vi "picoquant_read_buffer.vi"(8 "error in (no error)":errorcluster, 11 "picoquant_generic in":refnum<class "picoquant_generic.lvclass">) -> (0 "error out":errorcluster, 2 "new_data":u32[](array[numeric]), 3 "picoquant_generic out":refnum<class "picoquant_generic.lvclass">)   [LabVIEW 2015, in "picoquant_generic.lvclass"]
uses:
  picoquant_generic.lvclass
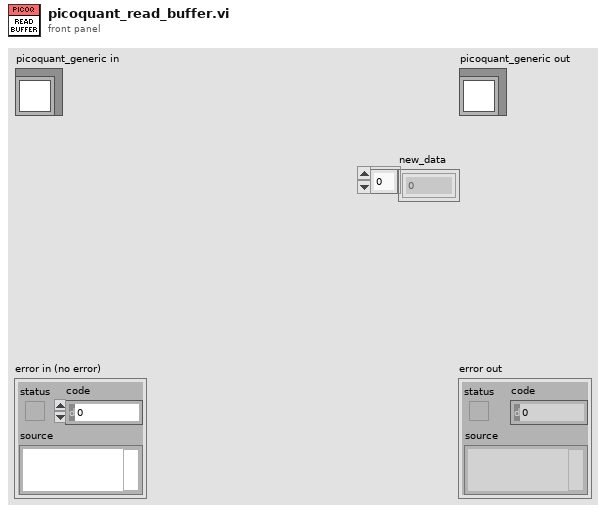
[diagram p1: front panel]
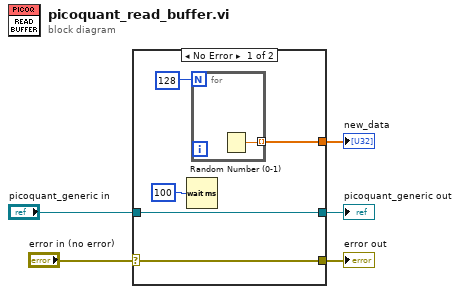
[diagram p0: block diagram]
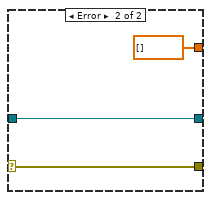
[diagram p2: hidden frame]
diagram:
  n1 = case shown="No Error" "error in (no error)" {
    selector: "error in (no error)" -> [w9 w14]
    tunnel: [w9 w14] -> w4
    tunnel: [w10 w13] -> w2
    tunnel: "picoquant_generic in" -> [w10 w13]
    tunnel: [w7 dbl[] []] -> w1
    frame No Error {
      n2 = Wait (ms)(milliseconds to wait=u32 100) -> ()  [unwired: 1 out]
      n3 = for {
        N: 128 -> [_]
        tunnel: [w11] -> w7 mode=indexing
        n4 = Random Number (0-1)() -> (number: 0 to 1=w11:dbl)
      }
    }
    frame Error {
    }
  }
  "error out" <- w4
  "picoquant_generic out" <- w2
  "new_data" <- w1
